vi "lift driver control.vi"(1 "Current Setpoint":dbl, 3 "Joystick Y":dbl) -> (0 "Setpoint":dbl)   [LabVIEW 2014]
uses:
  global variables/devrefs.vi
panel:
  # "Control the lift with PID setpoints instead of direct motor control"
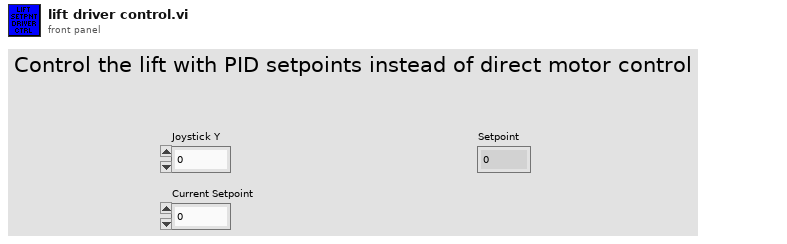
[diagram p1: front panel]
types:
  T1 = typedef "WPI_EncoderDevRef.ctl" = cluster{"DevStatus":errorcluster, "EncoderIndex":T2, "CounterIndex":T3, "DistancePerCount":dbl, "Decoding Type":T4}
  T2 = typedef "FPGA_EncoderIdx.ctl" = enum8{"Enc 0", "Enc 1", "Enc 2", "Enc 3", "Enc 4", "Enc 5", "Enc 6", "Enc 7", "Invalid"}
  T3 = typedef "FPGA_CounterCtrSystemIndex.ctl" = enum8{"Ctr 0", "Ctr 1", "Ctr 2", "Ctr 3", "Ctr 4", "Ctr 5", "Ctr 6", "Ctr 7", "Invalid"}
  T4 = typedef "WPI_EncoderType.ctl" = enum16{"1x", "2x", "4x"}
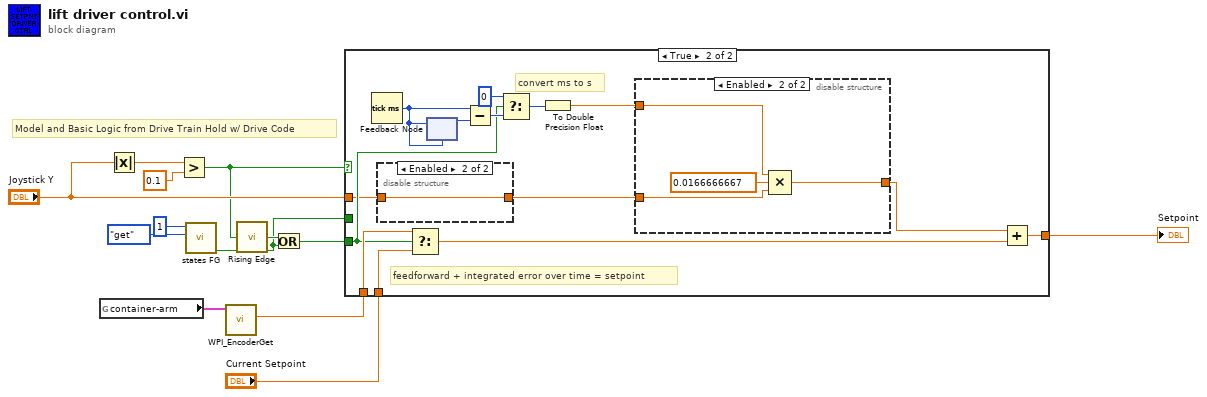
[diagram p0: block diagram]
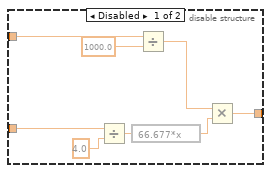
[diagram p4: hidden frame]
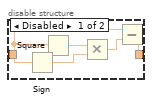
[diagram p5: hidden frame]
diagram:
  # "Model and Basic Logic from Drive Train Hold w/ Drive Code"
  n1 = global read "devrefs.vi" "container-arm"() -> (w3:T1)
  n2 = Absolute Value(x="Joystick Y") -> (abs(x)=w13:dbl)
  n3 = Greater?(x=w13, y=0.1) -> (0:w7:bool)
  n4 = call "states FG.vi"("menu (get)"=enum16{"set", "get"}."get", "Loop ID"=1) -> ("first call?"=w4:bool)  [unwired: 6 in, 3 out]
  n5 = call <vilib>:"WPI_EncoderGet.vi"("EncoderDevRef"=w3) -> ("Distance"=w6:dbl)  [unwired: 5 in, 5 out]
  n6 = call "Rising Edge.vi"("Input"=w7) -> ("Rising Edge"=w9:bool)
  n7 = Or(x=w9, y=w4) -> (x .or. y?=w5:bool)
  n8 = case shown="True" w7 {
    tunnel: "Joystick Y" -> [_ w26]
    tunnel: "Current Setpoint" -> [w17 w31]
    tunnel: w5 -> [_ w27]
    tunnel: w6 -> [w16 w30]
    tunnel: [w15 w24] -> w2
    tunnel: w4 -> [w14 _]
    frame False {
      n9 = case shown="False" w14 {
        tunnel: w17 -> [w18 _]
        tunnel: w16 -> [_ w19]
        tunnel: [w18 w19] -> w15
        frame False {
          # "and get it there if it isn't there"
          # "hold lift at current commanded location"
        }
        frame True {
          # "hold lift at encoder location"
        }
      }
    }
    frame True {
      # "feedforward + integrated error over time = setpoint"
      # "convert ms to s"
      n10 = Tick Count (ms)() -> (millisecond timer value=w21:u32)
      n11 = disable-structure shown="Enabled" {
        disable-tunnel: w26 -> [w50 w51]
        disable-tunnel: [w49 w51] -> w23
        frame Disabled {
          n12 = Sign(1:w50) -> (0:w47:dbl)
          n13 = Square(x=w50) -> (x^2=w48:dbl)
          n14 = Multiply(x=w48, y=w47) -> (x*y=w46:dbl)
          n15 = Subtract(x=w50, y=w46) -> (x-y=w49:dbl)
        }
        frame Enabled {
        }
      }
      n16 = Select(t=w30, s=w27, f=w31) -> (s? t:f=w25:dbl)
      n17 = feedback #1(w21) -> (w22:u32)
      n18 = feedback-in #1(w21) -> ()
      n19 = Subtract(x=w21, y=w22) -> (x-y=w32:u32)
      n20 = Select(t=u32 0, s=w27, f=w32) -> (s? t:f=w28:u32)
      n21 = To Double Precision Float(number=w28) -> (double precision float=w29:dbl)
      n22 = disable-structure shown="Enabled" {
        disable-tunnel: w29 -> [w41 w45]
        disable-tunnel: w23 -> [w37 w44]
        disable-tunnel: [w34 w42] -> w20
        frame Disabled {
          n23 = Divide(x=w37, y=4.0) -> (x/y=w36:dbl)
          n24 = expression code="66.677*x"(w36) -> (w35:dbl)
          n25 = Divide(x=w41, y=1000.0) -> (x/y=w39:dbl)
          n26 = Multiply(x=w39, y=w35) -> (x*y=w34:dbl)
        }
        frame Enabled {
          n27 = Compound Arithmetic op=MULTIPLY(w45, 0.0166666667 ("value"), w44) -> (w42:dbl)
        }
      }
      n28 = Add(x=w20, y=w25) -> (x+y=w24:dbl)
    }
  }
  "Setpoint" <- w2
